vi "LaserCal-Create Stimulus.vi"(0 "Stimulus":T2, 7 "Runtime State":T1={"AO Channels"=[], "Fs (Hz)"=100000.0, "Npts"=1, "conversion"=0.0}, 9 "Zero?":bool, 11 "error in (no error)":errorcluster) -> (8 "stimulus":dbl[][](array[numeric]), 10 "Duty Cycle":dbl, 15 "error out":errorcluster)   [LabVIEW 2015]
uses:
  Typedefs/LaserCal-Meter Stimulus.ctl
  Typedefs/LaserCal-Control Mode.ctl
  Typedefs/LaserCal-Meter Runtime State.ctl
  Signal Synthesis VIs/Waveform VIs/Pulse Train VIs/Pulse Train Params.ctl
  Signal Synthesis VIs/Waveform VIs/Pulse Train VIs/Pulse Polarity.ctl
  Signal Synthesis VIs/Waveform VIs/Pulse Train VIs/PT-Continuous State.ctl
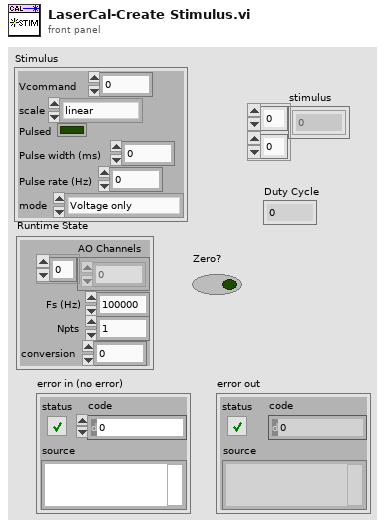
[diagram p1: front panel]
types:
  T1 = typedef "LaserCal-Meter Runtime State.ctl" = cluster{"AO Channels":i32[], "Fs (Hz)":dbl, "Npts":i32, "conversion":dbl}
  T2 = typedef "LaserCal-Meter Stimulus.ctl" = cluster{"Vcommand":dbl, "scale":enum16{"linear", "dB"}, "Pulsed":bool, "Pulse width (ms)":dbl, "Pulse rate (Hz)":dbl, "mode":T3}
  T3 = typedef "LaserCal-Control Mode.ctl" = enum16{"Voltage only", "Voltage + Enable"}
  T4 = typedef "Pulse Polarity.ctl" = enum16{"POS", "NEG", "POS-NEG", "NEG-POS"}
  T5 = typedef "Pulse Train Params.ctl" = cluster{"Pulse width (us)":dbl, "Pulse rate (Hz)":dbl, "Gap (ms)":dbl, "Polarity":T4, "PT State":T6, "Asynch":bool}
  T6 = typedef "PT-Continuous State.ctl" = cluster{"Template":dbl[], "Nperiod":i32, "Index":i32, "Pulse Rate (Hz)":dbl, "Phase (cycles)":dbl, "Noff":i32}
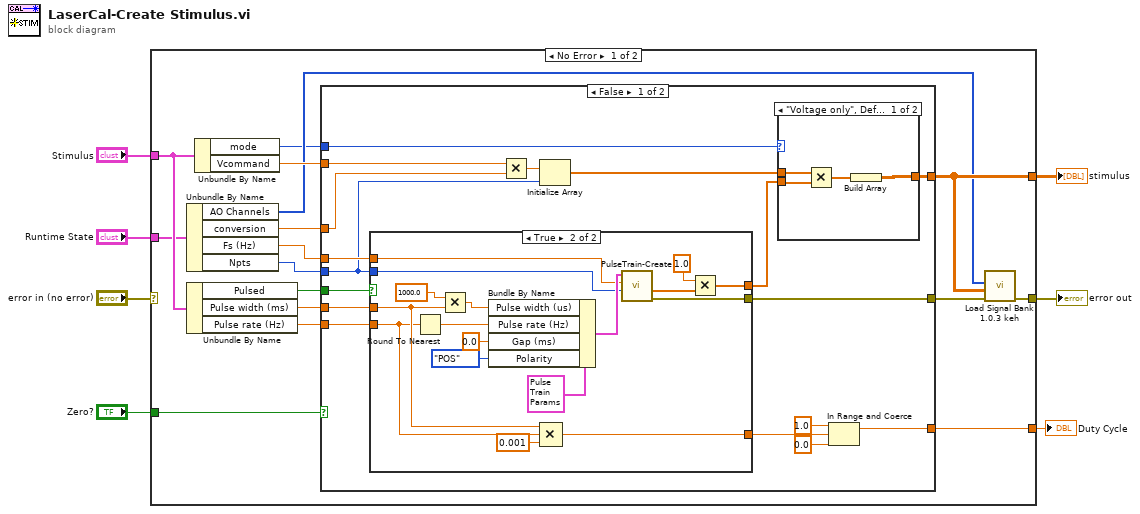
[diagram p0: block diagram]
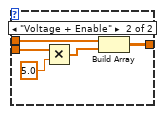
[diagram p2: hidden frame]
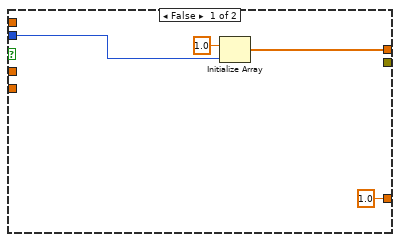
[diagram p3: hidden frame]
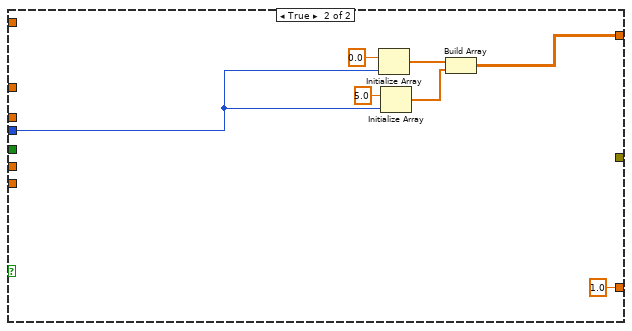
[diagram p4: hidden frame]
diagram:
  n1 = case shown="No Error" "error in (no error)" {
    selector: "error in (no error)" -> [_ w78]
    tunnel: "Stimulus" -> [w20 _]
    tunnel: [w16 _] -> w6
    tunnel: [w17 w78] -> w4
    tunnel: "Runtime State" -> [w15 _]
    tunnel: "Zero?" -> [w11 _]
    tunnel: [w9 _] -> w1
    frame No Error {
      n2 = Unbundle By Name(w15) -> ("AO Channels"=w13:i32[], "conversion"=w8:dbl, "Fs (Hz)"=w14:dbl, "Npts"=w12:i32)
      n3 = Unbundle By Name(w20) -> ("Pulsed"=w23:bool, "Pulse width (ms)"=w22:dbl, "Pulse rate (Hz)"=w21:dbl)
      n4 = Unbundle By Name(w20) -> ("mode"=w10:T3, "Vcommand"=w19:dbl)
      n5 = case shown="False" w11 {
        tunnel: w23 -> [w40 _]
        tunnel: w22 -> [w37 _]
        tunnel: w21 -> [w36 _]
        tunnel: w19 -> [w35 _]
        tunnel: [w34 _] -> w18
        tunnel: [w33 w73] -> w16
        tunnel: w14 -> [w32 _]
        tunnel: w12 -> [w31 w75]
        tunnel: w10 -> [w30 _]
        tunnel: [w26 1.0] -> w9
        tunnel: w8 -> [w28 _]
        frame False {
          n6 = case shown="True" w40 {
            tunnel: w36 -> [_ w56]
            tunnel: w37 -> [_ w57]
            tunnel: w32 -> [_ w64]
            tunnel: w31 -> [w53 w63]
            tunnel: [w51 w60] -> w39
            tunnel: [_ w61] -> w34
            tunnel: [1.0 w54] -> w27
            frame False {
              n7 = Initialize Array(1.0 ("element"), w53) -> (w51:dbl[])
            }
            frame True {
              n8 = Round To Nearest(number=w56) -> (nearest integer value=w62:dbl)
              n9 = Multiply(x=1000.0, y=w57) -> (x*y=w66:dbl)
              n10 = Bundle By Name(cluster=T5 {"Pulse width (us)"=0.0, "Pulse rate (Hz)"=0.0, "Gap (ms)"=0.0, "Polarity"=enum."POS", "PT State"={"Template"=[], "Nperiod"=0, "Index"=0, "Pulse Rate (Hz)"=0.0, "Phase (cycles)"=0.0, "Noff"=0}, "Asynch"=FALSE} ("Pulse Train Params"), "Pulse width (us)"=w66, "Pulse rate (Hz)"=w62, "Gap (ms)"=0.0, "Polarity"=Pulse_Polarity."POS") -> (w65:T5)
              n11 = Compound Arithmetic op=MULTIPLY(w57, w56, 0.001 ("value")) -> (w54:dbl)
              n12 = call "PulseTrain-Create.vi"("Npts"=w63, "Sampling Rate (Hz)"=w64, "Pulse Train Params"=w65) -> ("error out"=w61:errorcluster, "Waveform"=w58:dbl[])  [unwired: 5 in, 2 out]
              n13 = Multiply(x=1.0, y=w58) -> (x*y=w60:dbl[])
            }
          }
          n14 = Multiply(x=w35, y=w28) -> (x*y=w29:dbl)
          n15 = Initialize Array(w29, w31) -> (w38:dbl[])
          n16 = case shown="\"Voltage only\", Default" w30 {
            tunnel: w39 -> [w43 w49]
            tunnel: w38 -> [w44 w48]
            tunnel: [w41 w47] -> w33
            frame "Voltage only", Default {
              n17 = Multiply(x=w44, y=w43) -> (x*y=w42:dbl[])
              n18 = Build Array(w42) -> (w41:dbl[][])
            }
            frame "Voltage + Enable" {
              n19 = Multiply(x=w49, y=5.0) -> (x*y=w46:dbl[])
              n20 = Build Array(w48, w46) -> (w47:dbl[][])
            }
          }
          n21 = In Range and Coerce(upper limit=1.0, x=w27, lower limit=0.0) -> (coerced(x)=w26:dbl)  [unwired: 1 out]
        }
        frame True {
          n22 = Initialize Array(0.0 ("element"), w75) -> (w76:dbl[])
          n23 = Initialize Array(5.0 ("element"), w75) -> (w72:dbl[])
          n24 = Build Array(w76, w72) -> (w73:dbl[][])
        }
      }
      n25 = call "Load Signal Bank 1.0.3 keh.vi"("error in (no error)"=w18, "Input array"=w16, "Active AO Array"=w13) -> ("error out"=w17:errorcluster)  [unwired: 6 in, 2 out]
    }
    frame Error {
    }
  }
  "error out" <- w4
  "stimulus" <- w6
  "Duty Cycle" <- w1
